vi "界面3-试验结果.vi"() -> ()   [LabVIEW 2013]
panel:
  in  "要求值表格":bool
  out "Boolean":bool
  in  "reference":refnum<vi>
  in  "<--数据采集":bool
  in  "生成报告":bool
  in  "图像":bool
  in  "表格":bool
  in  "封面":bool
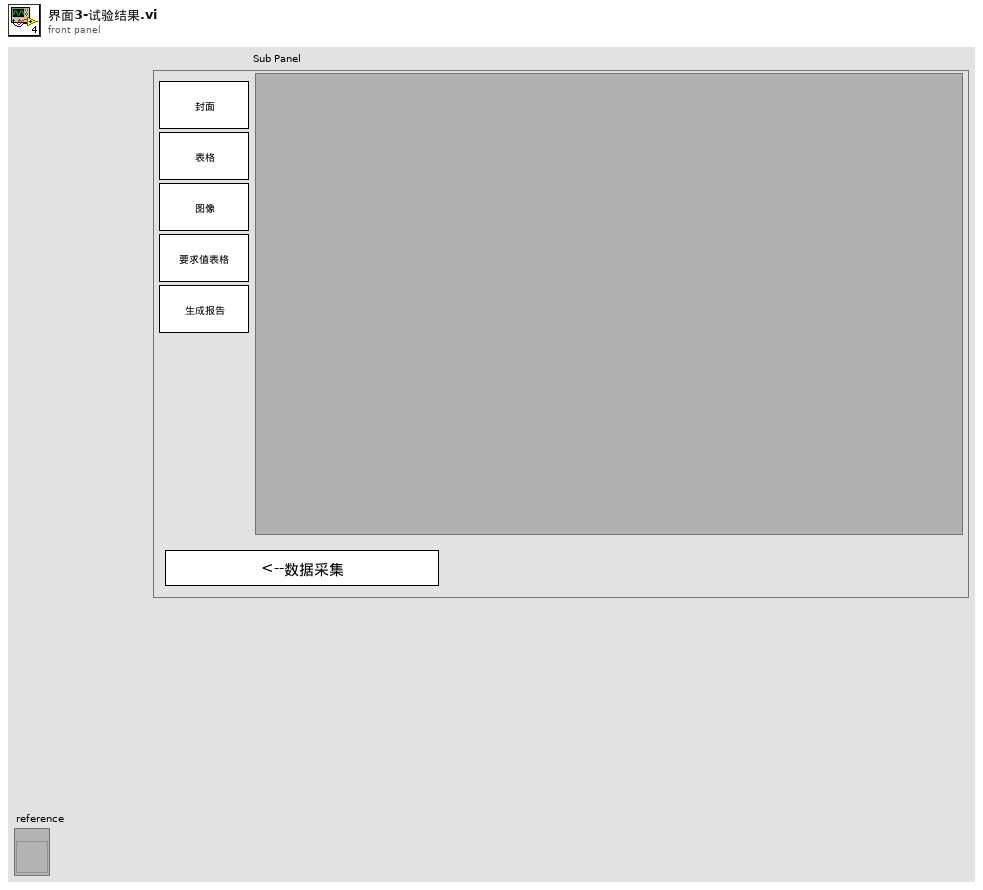
[diagram p1: front panel]
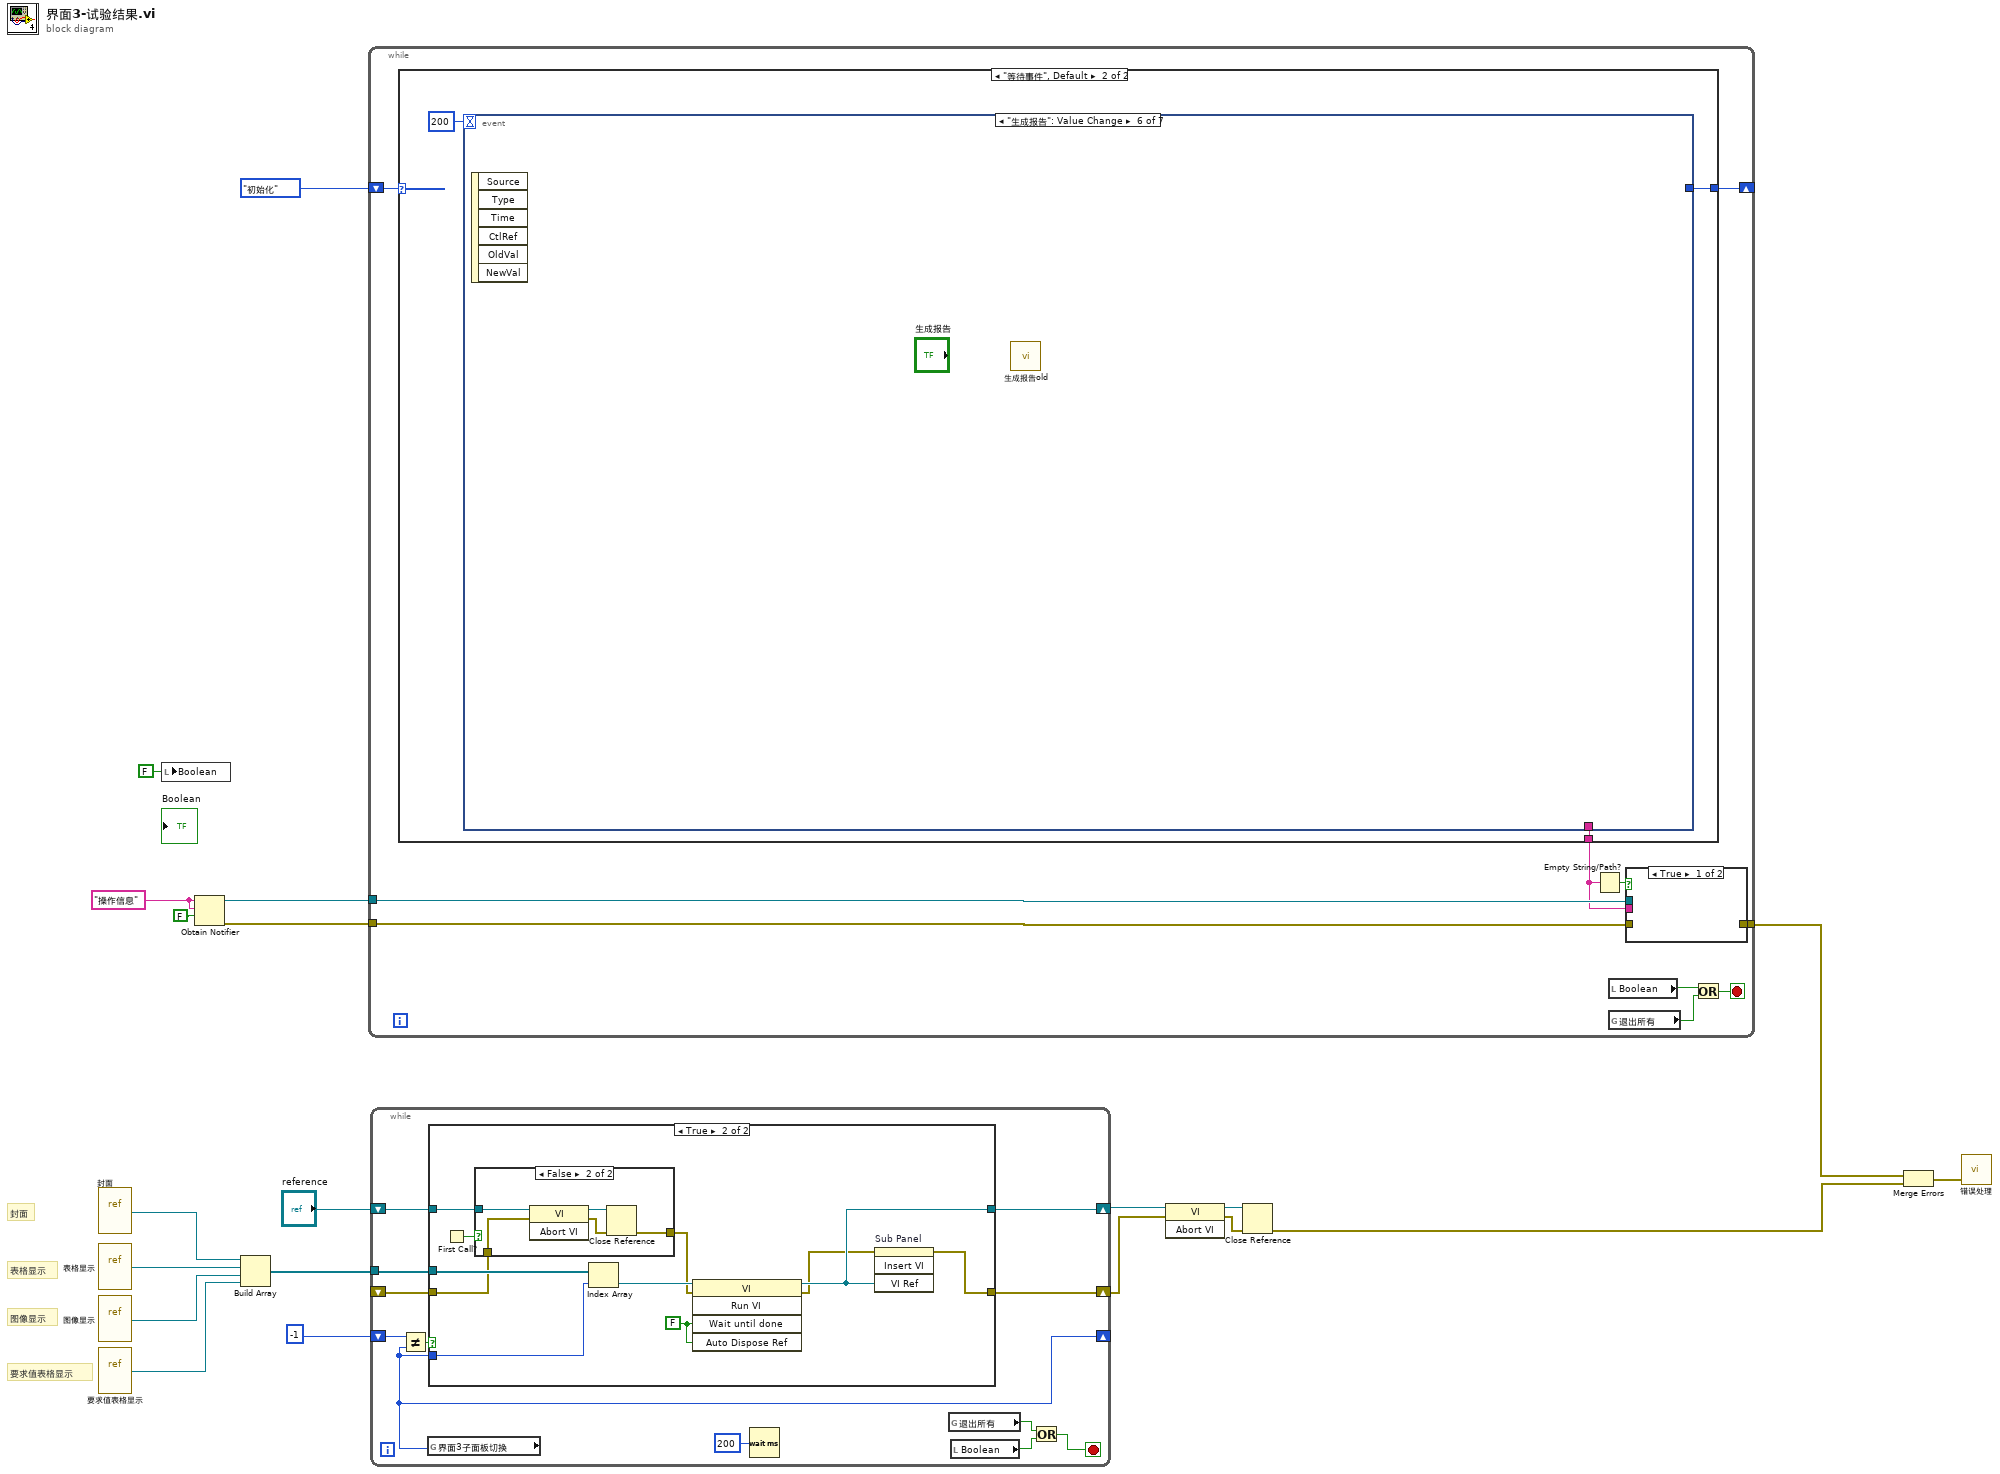
[diagram p0: block diagram]
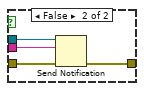
[diagram p4: hidden frame]
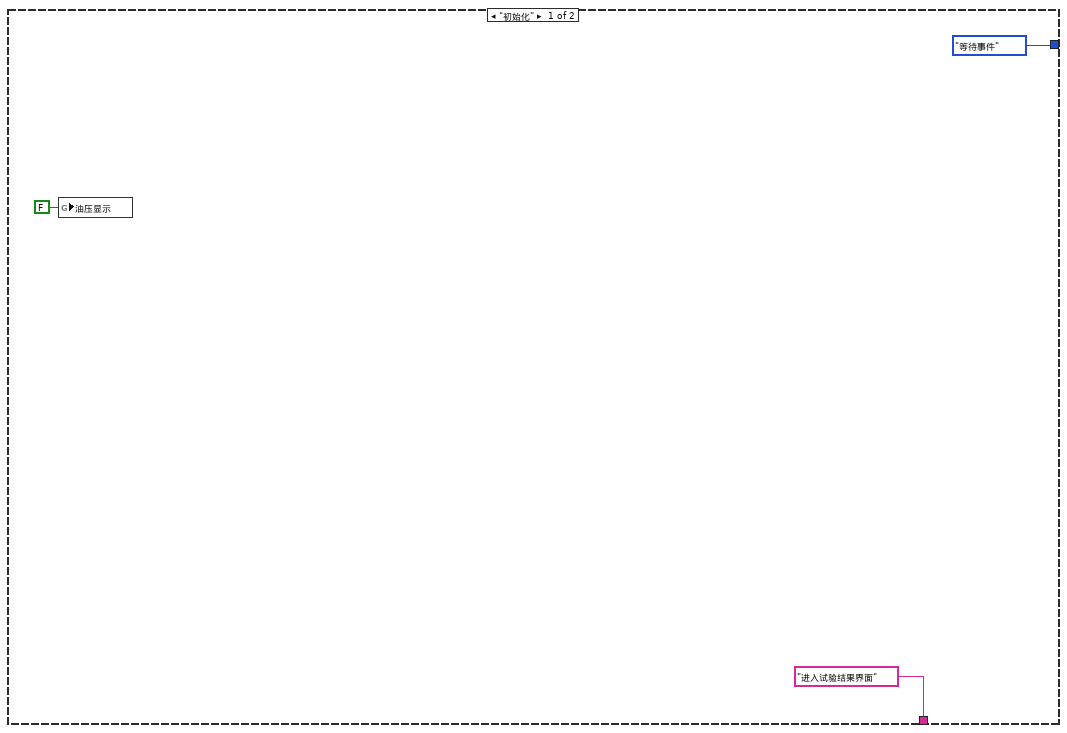
[diagram p5: hidden frame]
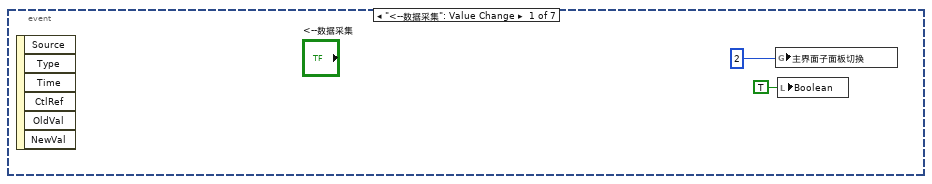
[diagram p6: hidden frame]
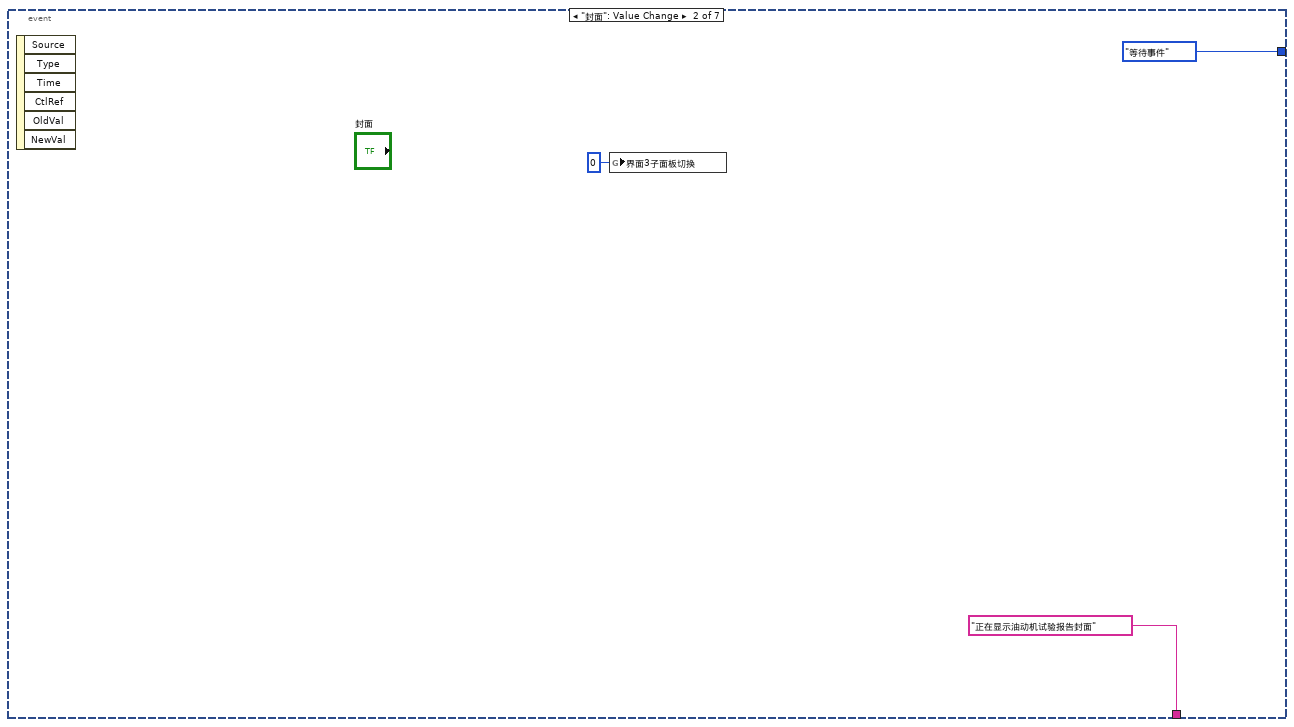
[diagram p7: hidden frame]
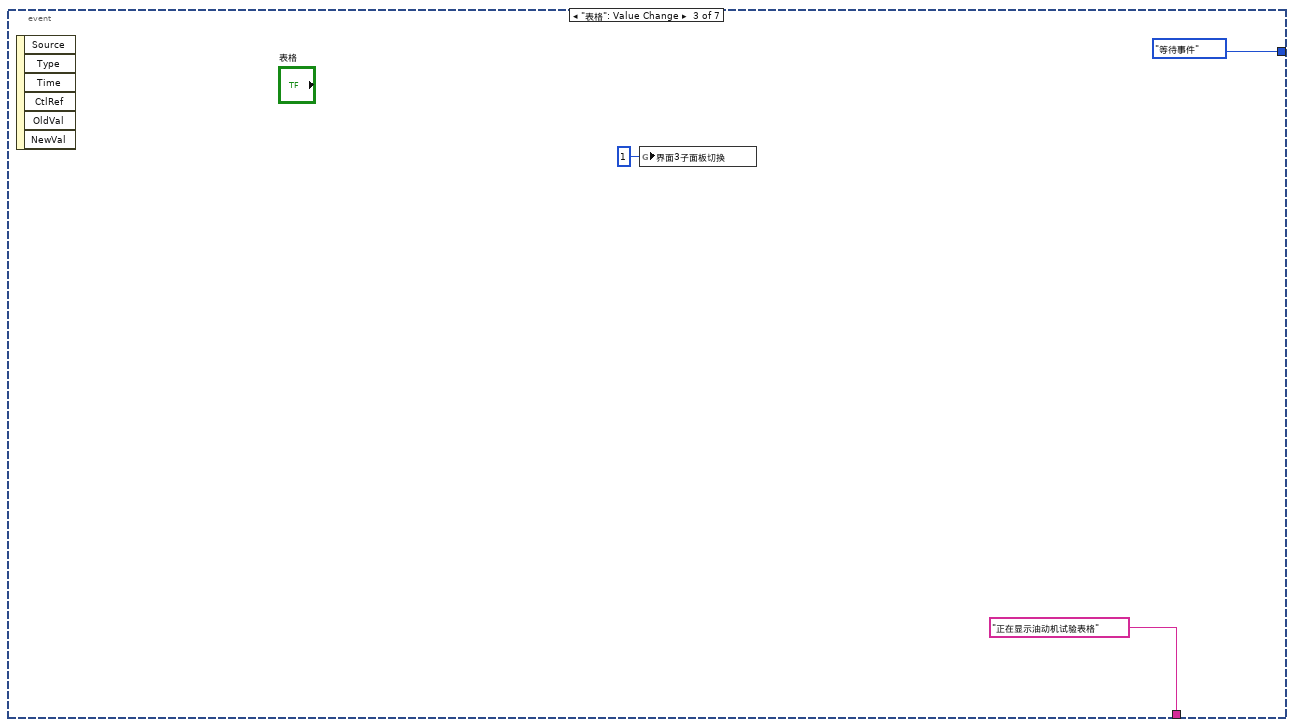
[diagram p8: hidden frame]
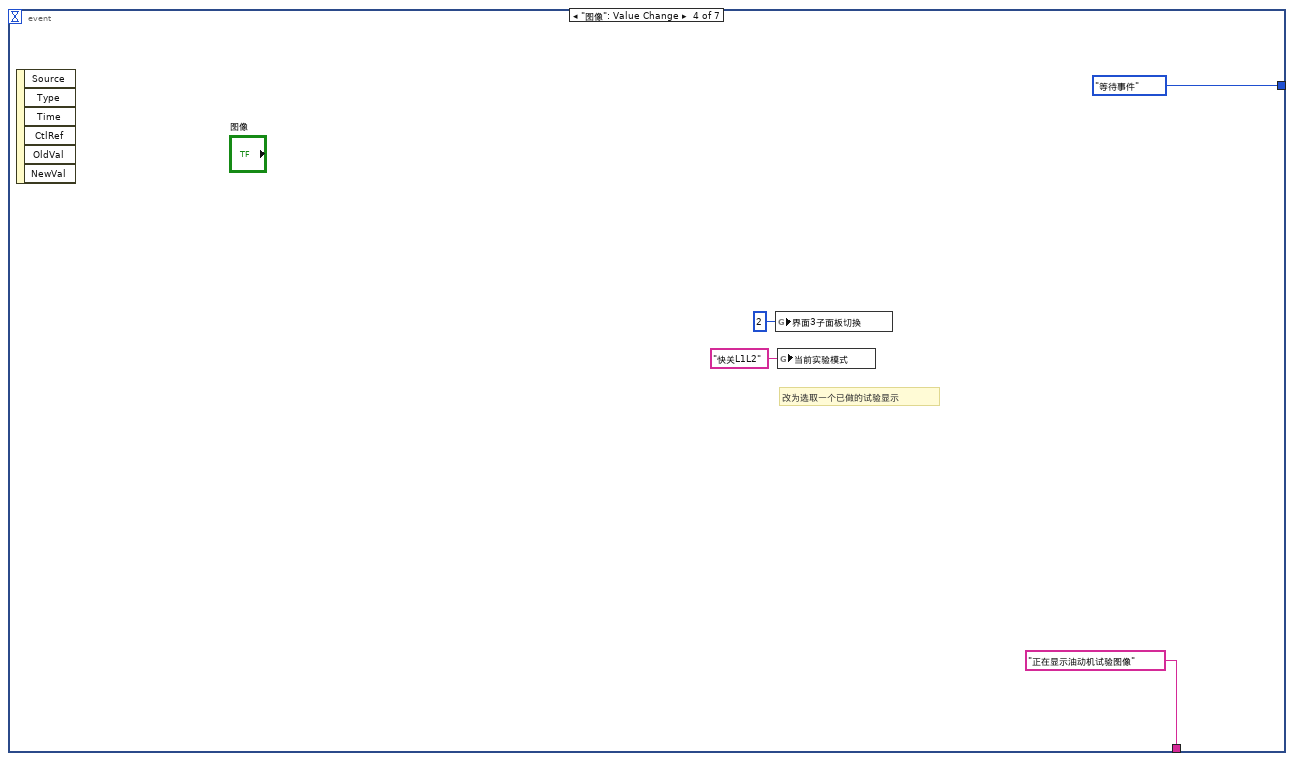
[diagram p9: hidden frame]
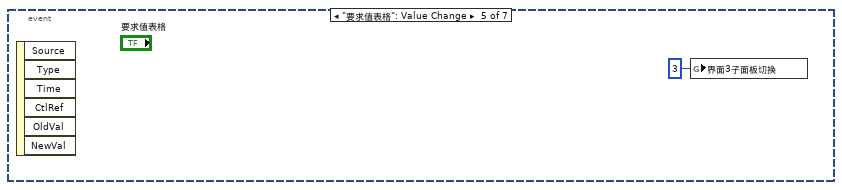
[diagram p10: hidden frame]
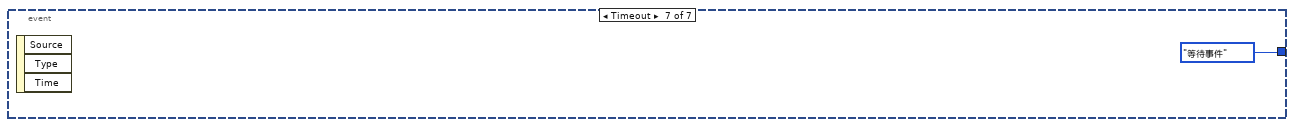
[diagram p11: hidden frame]
diagram:
  w19 = "操作信息"
  # "要求值表格显示"
  # "图像显示"
  # "封面"
  # "表格显示"
  n1 = vi-ref "封面.vi"() -> (w7:refnum<vi>)
  n2 = vi-ref "表格显示.vi"() -> (w8:refnum<vi>)
  n3 = vi-ref "图像显示.vi"() -> (w9:refnum<vi>)
  n4 = vi-ref "要求值表格显示.vi"() -> (w4:refnum<vi>)
  n5 = local write "Boolean"(FALSE ("Boolean")) -> ()
  n6 = Obtain Notifier(name (unnamed)=w19, notification data type=w19, create if not found? (T)=FALSE) -> (notifier out=w18:refnum<notifier>, error out=w17:errorcluster)  [unwired: 1 in, 1 out]
  n7 = Build Array(w7, w8, w9, w4) -> (w11:refnum<vi>[])
  n8 = while {
    shift-right: [w27] -> _
    shift-left: enum16{"初始化", "等待事件"}."初始化" -> [w30]
    tunnel: w18 -> [w29]
    tunnel: w17 -> [w28]
    tunnel: [w21] -> w3
    stop <- w26 stop-if-true
    n9 = case shown="\"等待事件\", Default" w30 {
      tunnel: ["进入试验结果界面" w39] -> w22
      tunnel: [enum16{"初始化", "等待事件", "表格", "图像显示"}."等待事件" w40] -> w27
      frame "初始化" {
        n10 = global write "油压显示.vi" "油压显示"(FALSE ("油压显示")) -> ()
      }
      frame "等待事件", Default {
        n11 = event shown="[5] \"生成报告\": Value Change" {
          selector: _ -> [_ _ _ _ _ _ _]
          dyn-events: _ -> [_ _ _ _ _ _ _]
          timeout: 200 -> [_ _ _ _ _ _ _]
          tunnel: [_ enum16{"初始化", "等待事件"}."等待事件" enum16{"初始化", "等待事件"}."等待事件" enum16{"初始化", "等待事件"}."等待事件" _ _ enum16{"初始化", "等待事件"}."等待事件"] -> w40
          tunnel: [_ "正在显示油动机试验报告封面" "正在显示油动机试验表格" "正在显示油动机试验图像" _ _ _] -> w39
          event "<--数据采集": Value Change {
            n12 = event-data() -> ()  [unwired: 1 in, 6 out]
            n13 = global write "主界面子面板切换.vi" "主界面子面板切换"(2) -> ()
            n14 = local write "Boolean"(TRUE ("Boolean")) -> ()
          }
          event "封面": Value Change {
            n15 = event-data() -> ()  [unwired: 1 in, 6 out]
            n16 = global write "界面3子面板切换.vi" "界面3子面板切换"(0 ("界面3子面板切换")) -> ()
          }
          event "表格": Value Change {
            n17 = event-data() -> ()  [unwired: 1 in, 6 out]
            n18 = global write "界面3子面板切换.vi" "界面3子面板切换"(1 ("界面3子面板切换")) -> ()
          }
          event "图像": Value Change {
            # "改为选取一个已做的试验显示"
            n19 = event-data() -> ()  [unwired: 1 in, 6 out]
            n20 = global write "界面3子面板切换.vi" "界面3子面板切换"(2 ("界面3子面板切换")) -> ()
            n21 = global write "当前实验模式.vi" "当前实验模式"("快关L1L2" ("当前实验模式")) -> ()
          }
          event "要求值表格": Value Change {
            n22 = event-data() -> ()  [unwired: 1 in, 6 out]
            n23 = global write "界面3子面板切换.vi" "界面3子面板切换"(3 ("界面3子面板切换")) -> ()
          }
          event "生成报告": Value Change {
            n24 = event-data() -> ()  [unwired: 1 in, 6 out]
            n25 = call "生成报告old.vi"() -> ()  [unwired: 12 in]
          }
          event Timeout {
            n26 = event-data() -> ()  [unwired: 1 in, 3 out]
          }
        }
      }
    }
    n27 = Empty String/Path?(string/path=w22) -> (empty?=w23:bool)
    n28 = local read "Boolean"() -> (w25:bool)
    n29 = global read "退出所有.vi" "退出所有"() -> (w24:bool)
    n30 = case shown="True" w23 {
      tunnel: w29 -> [_ w34]
      tunnel: w28 -> [_ w33]
      tunnel: w22 -> [_ w32]
      tunnel: [_ w31] -> w21
      frame True {
      }
      frame False {
        n31 = Send Notification(notification=w32, notifier=w34, error in (no error)=w33) -> (error out=w31:errorcluster)  [unwired: 1 out]
      }
    }
    n32 = Or(x=w25, y=w24) -> (x .or. y?=w26:bool)
  }
  n33 = while {
    tunnel: w11 -> [w66]
    shift-right: [w64] -> w5
    shift-left: _ -> [w65]
    shift-right: [w58] -> _
    shift-left: -1 -> [w62]
    shift-right: [w60] -> w15
    shift-left: "reference" -> [w59]
    stop <- w57 stop-if-true
    n34 = global read "界面3子面板切换.vi" "界面3子面板切换"() -> (w58:i32)
    n35 = Not Equal?(x=w62, y=w58) -> (x != y?=w61:bool)
    n36 = case shown="True" w61 {
      tunnel: w66 -> [_ w79]
      tunnel: w65 -> [w68 w70]
      tunnel: [w68 w71] -> w64
      tunnel: w58 -> [_ w76]
      tunnel: [w67 w73] -> w60
      tunnel: w59 -> [w67 w74]
      frame False {
      }
      frame True {
        w77 = FALSE
        n37 = First Call?() -> (First Call?: T/F=w75:bool)
        n38 = case shown="False" w75 {
          tunnel: w74 -> [_ w82]
          tunnel: w70 -> [_ w81]
          tunnel: [_ w80] -> w69
          frame True {
          }
          frame False {
            n39 = invoke class="VI" method="Abort VI"(reference=w82, error in=w81) -> (reference out=w84:refnum<vi>, error out=w83:errorcluster)  [unwired: 1 in, 1 out]
            n40 = Close Reference(reference=w84, error in (no error)=w83) -> (error out=w80:errorcluster)
          }
        }
        n41 = Index Array(array=w79, index=w76) -> (element=w78:refnum<vi>)
        n42 = invoke class="VI" method="Run VI"(reference=w78, error in=w69, "Wait until done"=w77, "Auto Dispose Ref"=w77) -> (reference out=w73:refnum<vi>, error out=w72:errorcluster)  [unwired: 1 in, 3 out]
        n43 = invoke on="Sub Panel" class="SubPanel" method="Insert VI"(error in=w72, "VI Ref"=w73) -> (error out=w71:errorcluster)  [unwired: 2 in, 3 out]
      }
    }
    n44 = Wait (ms)(milliseconds to wait=u32 200) -> ()  [unwired: 1 out]
    n45 = global read "退出所有.vi" "退出所有"() -> (w56:bool)
    n46 = local read "Boolean"() -> (w55:bool)
    n47 = Or(x=w56, y=w55) -> (x .or. y?=w57:bool)
  }
  n48 = invoke class="VI" method="Abort VI"(reference=w15, error in=w5) -> (reference out=w13:refnum<vi>, error out=w14:errorcluster)  [unwired: 1 in, 1 out]
  n49 = Close Reference(reference=w13, error in (no error)=w14) -> (error out=w2:errorcluster)
  n50 = Merge Errors(w3, w2) -> (w1:errorcluster)
  n51 = call "错误处理.vi"("error in (no error)"=w1) -> ()  [unwired: 2 in]
